vi "test-traj-generate-8-way.vi"() -> ()   [LabVIEW 2019]
uses:
  <vilib>/Rock Robotics/WPI/ThirdParty/JAS_Junk/TrajLib/WAYPOINTS.ctl
  <vilib>/Rock Robotics/WPI/ThirdParty/JAS_Junk/TrajLib/TRANSLATION2D.ctl
  <vilib>/Rock Robotics/WPI/ThirdParty/JAS_Junk/TrajLib/TRAJECTORY.ctl
  <vilib>/Rock Robotics/WPI/ThirdParty/JAS_Junk/TrajLib/TRAJ_STATE.ctl
  <vilib>/Rock Robotics/WPI/ThirdParty/JAS_Junk/TrajLib/POSE2D.ctl
  <vilib>/Rock Robotics/WPI/ThirdParty/JAS_Junk/TrajLib/ROTATION2D.ctl
  <vilib>/Rock Robotics/WPI/ThirdParty/JAS_Junk/TrajLib/X_Y_HEADING.ctl
  <vilib>/Rock Robotics/WPI/ThirdParty/JAS_Junk/TrajLib/SPLINE.ctl
  <vilib>/Analysis/Matrix/Datatypes/RealMatrix.ctl
  <vilib>/Rock Robotics/WPI/ThirdParty/JAS_Junk/TrajLib/POSEwCURVATURE.ctl
  <vilib>/Rock Robotics/WPI/ThirdParty/JAS_Junk/TrajLib/TRAJ_CONFIG.ctl
  <vilib>/Rock Robotics/WPI/ThirdParty/JAS_Junk/TrajLib/TRAJ_CONSTRAINT_DIIF_DRIVE_KINEMATICS.ctl
  <vilib>/Rock Robotics/WPI/ThirdParty/JAS_Junk/TrajLib/DIFF_DRIVE_KINEMATICS.ctl
  <vilib>/Rock Robotics/WPI/ThirdParty/JAS_Junk/TrajLib/TRAJ_CONSTRAINT_CENTRIPETAL_ACCEL.ctl
  <vilib>/Rock Robotics/WPI/ThirdParty/JAS_Junk/TrajLib/TRAJ_CONSTRAINT_SWERVE_DRIVE_KINEMATICS.ctl
  <vilib>/Rock Robotics/WPI/ThirdParty/JAS_Junk/TrajLib/SWERVE_DRIVE_KINEMATICS.ctl
  <vilib>/Rock Robotics/WPI/ThirdParty/JAS_Junk/TrajLib/TRAJ_CONSTRAINT_DIIF_DRIVE_VOLTAGE.ctl
  <vilib>/Rock Robotics/WPI/ThirdParty/JAS_Junk/TrajLib/SIMPLE_MOTOR_FF.ctl
  <vilib>/Rock Robotics/WPI/ThirdParty/JAS_Junk/TrajLib/TRAJ_CONSTRAINT_MECA_DRIVE_KINEMATICS.ctl
  <vilib>/Rock Robotics/WPI/ThirdParty/JAS_Junk/TrajLib/MECA_DRIVE_KINEMATICS.ctl
  <vilib>/Rock Robotics/WPI/ThirdParty/JAS_Junk/TrajLib/UTIL_WAYPOINT.ctl
  <vilib>/Rock Robotics/SystemInterfaces/NetworkCommunication/NetComm_UsageReport_report.vi
  <vilib>/Rock Robotics/WPI/ThirdParty/JAS_Junk/TrajLib/DiffDriveKinematicsConstraint_New.vi
  <vilib>/Rock Robotics/WPI/ThirdParty/JAS_Junk/TrajLib/CentripetalAccelConstraint_New.vi
  <vilib>/Rock Robotics/WPI/ThirdParty/JAS_Junk/TrajLib/Rotation_CreateAngle.vi
  <vilib>/Rock Robotics/WPI/ThirdParty/JAS_Junk/TrajLib/Translation_Create.vi
  <vilib>/Rock Robotics/WPI/ThirdParty/JAS_Junk/TrajLib/Util_LibraryGlobals.vi
  <vilib>/Rock Robotics/WPI/ThirdParty/JAS_Junk/TrajLib/Trajectory_Library.lvlib
  <vilib>/Analysis/Matrix/NI_Matrix.lvlib
panel:
  in  "Tab Control":T1(tab)
  in  "Interior WAYPOINTS":T2=[{"X"=1.5, "Y"=1.5}, {"X"=0.0, "Y"=0.0}, {"X"=-1.5, "Y"=-1.5}, {"X"=-3.0, "Y"=0.0}, {"X"=-1.5, "Y"=1.5}, {"X"=0.0, "Y"=0.0}, {"X"=1.5, "Y"=-1.5}]
  in  "Initial_Position":T4={"X"=3.0, "Y"=0.0, "Heading"=1.571}
  in  "Ending_Position":T4={"X"=3.0, "Y"=0.0, "Heading"=1.571}
  out "splines":T5[](array[typedef])
  out "ArrayPoseWithCurvature":T7[](array[typedef])
  out "PoseCSize":i32
  out "error out 2":errorcluster
  in  "MaxVelocity":dbl=2.0 format="%17.4f"
  in  "MaxAcceleration":dbl=1.3 format="%17.4f"
  in  "TrackWidth_Meters":dbl=0.66 format="%20.4f"
  in  "Max Cent Accel":dbl=1.0 format="%20.4f"
  out "outTRAJECTORY_CONFIG":T10={"MaxVelocity"=0.0, "Max Acceleration"=0.0, "StartVelocity"=0.0, "End Velocity"=0.0, "Reversed"=FALSE, "DiffDrKineConstntDefined"=FALSE, "CentAcellConstntDefined"=FALSE, "DiffDrVoltConstntDefined"=FALSE, "DIFF_DRIVE_KINE_CONSTRAINT"={"Max Speed (M/S)"=0.0, "DIFF_DRIVE_KINEMATICS"={"TrackWidth_Meters"=0.0}}, "CENTRIPETAL_ACCEL_CONSTRAINT"={"Max Cent Accel"=0.0}, "SwerveDrKineConstntDefined"=FALSE, "SWERVE_DRIVE_KINE_CONSTRAINT"={"Max Speed (M/S)"=0.0, "SwerveKinematics"={"NumModules"=0, "InverseKinematics"=[], "ForwardKinematics"=[], "Modules"=[], "PrevCoR"={"X"=0.0, "Y"=0.0}}}, "DIFF_DRIVE_VOLTAGE_CONSTRAINT"={"Max Voltage"=0.0, "DIFF_DRIVE_KINEMATICS"={"TrackWidth_Meters"=0.0}, "SIMPLE_MOTOR_FF"={"Ks"=0.0, "Kv"=0.0, "Ka"=0.0}}, "MECANUM_DRIVE_KINE_CONSTRAINT"={"Max Speed (M/S)"=0.0, "MECA_DRIVE_KINEMATICS"={"FrontLeft"={"X"=0.0, "Y"=0.0}, "FrontRight"={"X"=0.0, "Y"=0.0}, "RearLeft"={"X"=0.0, "Y"=0.0}, "RearRight"={"X"=0.0, "Y"=0.0}, "InverseKinematics"=[[0.0, 1.0, -1.0, 0.0], [0.0, 1.0, 1.0, 0.0], [0.0, 1.0, 1.0, 0.0], [0.0, 1.0, -1.0, 0.0]], "ForwardKinematics"=[[0.0, 1.0, -1.0, 0.0], [0.0, 1.0, 1.0, 0.0], [0.0, 1.0, 1.0, 0.0], [0.0, 1.0, -1.0, 0.0]], "PrevCoR"={"X"=0.0, "Y"=0.0}}}, "MecanumDrKineConstntDefined"=FALSE} {"MECANUM_DRIVE_KINE_CONSTRAINT"."MECA_DRIVE_KINEMATICS"."PrevCoR"."Y" format="%14.3f"; "MECANUM_DRIVE_KINE_CONSTRAINT"."MECA_DRIVE_KINEMATICS"."PrevCoR"."X" format="%14.3f"; "MECANUM_DRIVE_KINE_CONSTRAINT"."MECA_DRIVE_KINEMATICS"."RearRight"."Y" format="%14.3f"; "MECANUM_DRIVE_KINE_CONSTRAINT"."MECA_DRIVE_KINEMATICS"."RearRight"."X" format="%14.3f"; "MECANUM_DRIVE_KINE_CONSTRAINT"."MECA_DRIVE_KINEMATICS"."RearLeft"."Y" format="%14.3f"; "MECANUM_DRIVE_KINE_CONSTRAINT"."MECA_DRIVE_KINEMATICS"."RearLeft"."X" format="%14.3f"; "MECANUM_DRIVE_KINE_CONSTRAINT"."MECA_DRIVE_KINEMATICS"."FrontRight"."Y" format="%14.3f"; "MECANUM_DRIVE_KINE_CONSTRAINT"."MECA_DRIVE_KINEMATICS"."FrontRight"."X" format="%14.3f"; "MECANUM_DRIVE_KINE_CONSTRAINT"."MECA_DRIVE_KINEMATICS"."FrontLeft"."Y" format="%14.3f"; "MECANUM_DRIVE_KINE_CONSTRAINT"."MECA_DRIVE_KINEMATICS"."FrontLeft"."X" format="%14.3f"; "MECANUM_DRIVE_KINE_CONSTRAINT"."Max Speed (M/S)" format="%20.4f"; "DIFF_DRIVE_VOLTAGE_CONSTRAINT"."SIMPLE_MOTOR_FF"."Ka" format="%13.4f"; "DIFF_DRIVE_VOLTAGE_CONSTRAINT"."SIMPLE_MOTOR_FF"."Kv" format="%13.4f"; "DIFF_DRIVE_VOLTAGE_CONSTRAINT"."SIMPLE_MOTOR_FF"."Ks" format="%13.4f"; "DIFF_DRIVE_VOLTAGE_CONSTRAINT"."DIFF_DRIVE_KINEMATICS"."TrackWidth_Meters" format="%20.4f"; "DIFF_DRIVE_VOLTAGE_CONSTRAINT"."Max Voltage" format="%20.4f"; "SWERVE_DRIVE_KINE_CONSTRAINT"."SwerveKinematics"."PrevCoR"."Y" format="%14.3f"; "SWERVE_DRIVE_KINE_CONSTRAINT"."SwerveKinematics"."PrevCoR"."X" format="%14.3f"; "SWERVE_DRIVE_KINE_CONSTRAINT"."SwerveKinematics"."Modules"."Y" format="%14.3f"; "SWERVE_DRIVE_KINE_CONSTRAINT"."SwerveKinematics"."Modules"."X" format="%14.3f"; "SWERVE_DRIVE_KINE_CONSTRAINT"."Max Speed (M/S)" format="%20.4f"; "CENTRIPETAL_ACCEL_CONSTRAINT"."Max Cent Accel" format="%20.4f"; "DIFF_DRIVE_KINE_CONSTRAINT"."DIFF_DRIVE_KINEMATICS"."TrackWidth_Meters" format="%20.4f"; "DIFF_DRIVE_KINE_CONSTRAINT"."Max Speed (M/S)" format="%20.4f"; "End Velocity" format="%20.4f"; "StartVelocity" format="%20.4f"; "Max Acceleration" format="%20.4f"; "MaxVelocity" format="%20.4f"}
  out "TRAJECTORY":T20 {"TotalTImeSecs" format="%20.3f"}
  out "size(s)":i32
  out "error out":errorcluster
  out "read Traj":errorcluster
  out "readTRAJECTORY":T20 {"TotalTImeSecs" format="%20.3f"}
  out "size(s) 2":i32
  out "file write error":errorcluster
  out "appended path":path
  out "XY Graph":cluster{dbl[], dbl[]}(graph)
  out "Position":cluster{dbl[], dbl[]}(graph)
  out "Time":dbl
  in  "STEP":bool
  out "XY Graph 2":cluster{dbl[], dbl[]}(graph)
  out "TimeSeconds":dbl
  out "OutputTRAJ_STATE":T21={"TimeSeconds"=0.0, "Velocity"=0.0, "Acceleration"=0.0, "POSE"={"TRANSLATION"={"X"=0.0, "Y"=0.0}, "ROTATION"={"VALUE"=0.0, "COS"=1.0, "SIN"=0.0}}, "Curvature"=0.0}
  in  "CONT":bool
  out "Done":bool
  # "ARRAY OF OTHER\nCONSTRAINTS \nGOES HERE.."
  # "Single step\nthrough \ntrajectory"
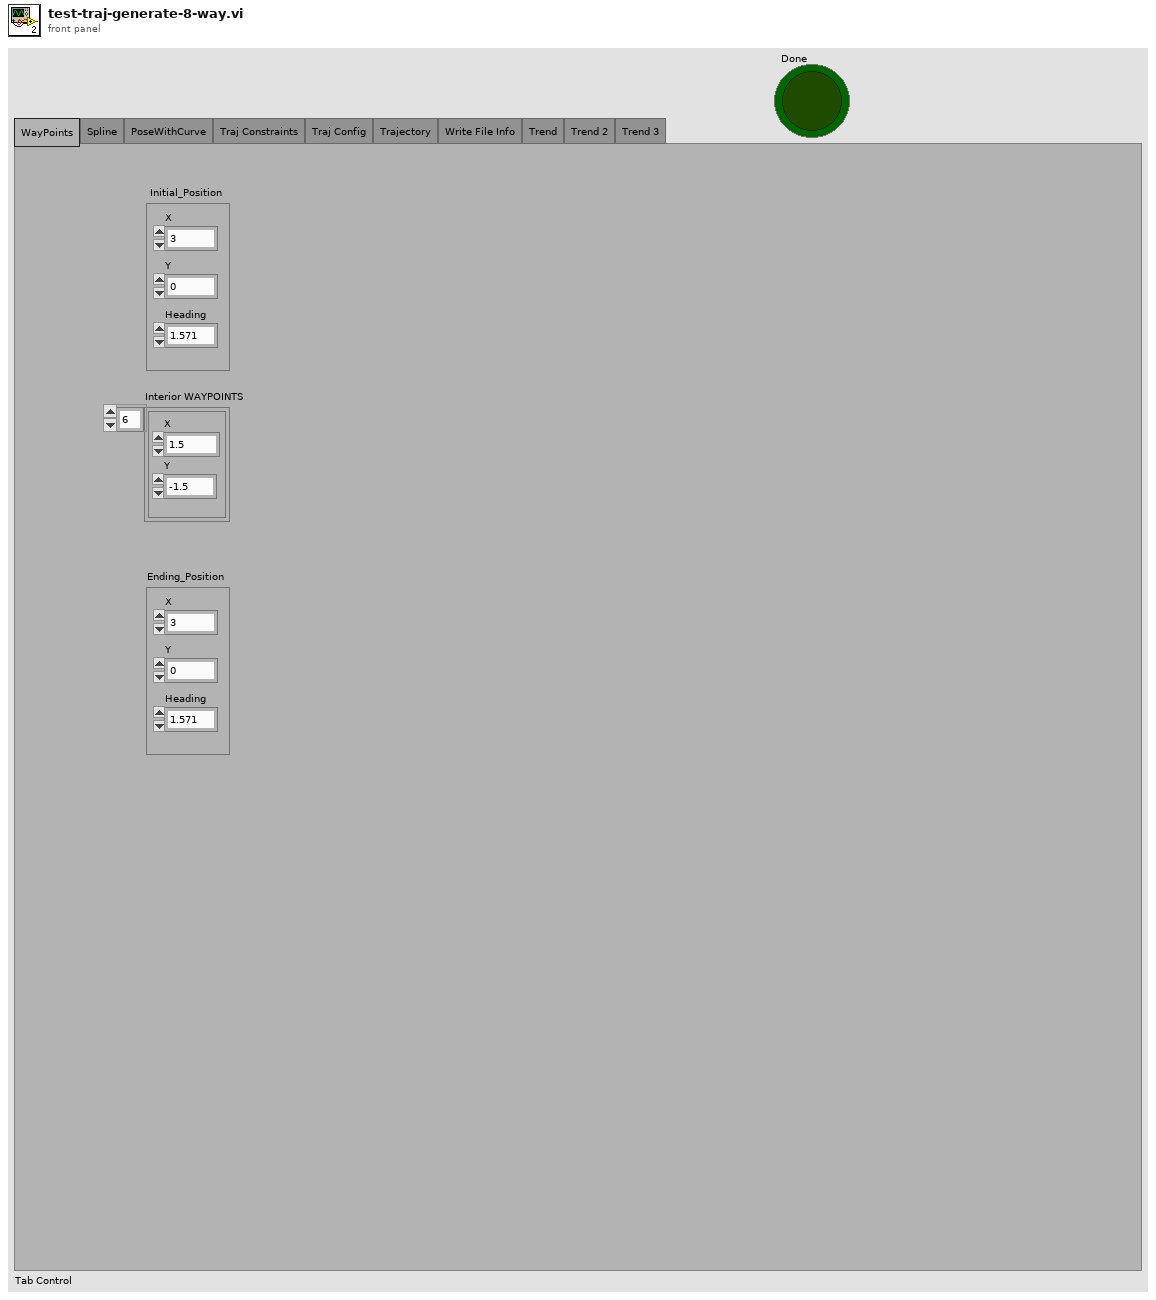
[diagram p1: front panel]
types:
  T1 = enum32{"WayPoints", "Spline", "PoseWithCurve", "Traj Constraints", "Traj Config", "Trajectory", "Write File Info", "Trend", "Trend 2", "Trend 3"}
  T2 = typedef "Trajectory_Library.lvlib/WAYPOINTS.ctl" = T3[]
  T3 = typedef "Trajectory_Library.lvlib/TRANSLATION2D.ctl" = cluster{"X":dbl, "Y":dbl}
  T4 = typedef "Trajectory_Library.lvlib/X_Y_HEADING.ctl" = cluster{"X":dbl, "Y":dbl, "Heading":dbl}
  T5 = typedef "Trajectory_Library.lvlib/SPLINE.ctl" = cluster{"Degree":i32, "Coefficients":T6}
  T6 = typedef "NI_Matrix.lvlib/RealMatrix.ctl" = dbl[][]
  T7 = typedef "Trajectory_Library.lvlib/POSEwCURVATURE.ctl" = cluster{"CURVATURE":dbl, "POSE":T8}
  T8 = typedef "Trajectory_Library.lvlib/POSE2D.ctl" = cluster{"TRANSLATION":T3, "ROTATION":T9}
  T9 = typedef "Trajectory_Library.lvlib/ROTATION2D.ctl" = cluster{"VALUE":dbl, "COS":dbl, "SIN":dbl}
  T10 = typedef "Trajectory_Library.lvlib/TRAJ_CONFIG.ctl" = cluster{"MaxVelocity":dbl, "Max Acceleration":dbl, "StartVelocity":dbl, "End Velocity":dbl, "Reversed":bool, "DiffDrKineConstntDefined":bool, "CentAcellConstntDefined":bool, "DiffDrVoltConstntDefined":bool, "DIFF_DRIVE_KINE_CONSTRAINT":T11, "CENTRIPETAL_ACCEL_CONSTRAINT":T13, "SwerveDrKineConstntDefined":bool, "SWERVE_DRIVE_KINE_CONSTRAINT":T14, "DIFF_DRIVE_VOLTAGE_CONSTRAINT":T16, "MECANUM_DRIVE_KINE_CONSTRAINT":T18, "MecanumDrKineConstntDefined":bool}
  T11 = typedef "Trajectory_Library.lvlib/TRAJ_CONSTRAINT_DIIF_DRIVE_KINEMATICS.ctl" = cluster{"Max Speed (M/S)":dbl, "DIFF_DRIVE_KINEMATICS":T12}
  T12 = typedef "Trajectory_Library.lvlib/DIFF_DRIVE_KINEMATICS.ctl" = cluster{"TrackWidth_Meters":dbl}
  T13 = typedef "Trajectory_Library.lvlib/TRAJ_CONSTRAINT_CENTRIPETAL_ACCEL.ctl" = cluster{"Max Cent Accel":dbl}
  T14 = typedef "Trajectory_Library.lvlib/TRAJ_CONSTRAINT_SWERVE_DRIVE_KINEMATICS.ctl" = cluster{"Max Speed (M/S)":dbl, "SwerveKinematics":T15}
  T15 = typedef "Trajectory_Library.lvlib/SWERVE_DRIVE_KINEMATICS.ctl" = cluster{"NumModules":i32, "InverseKinematics":T6, "ForwardKinematics":T6, "Modules":T3[], "PrevCoR":T3}
  T16 = typedef "Trajectory_Library.lvlib/TRAJ_CONSTRAINT_DIIF_DRIVE_VOLTAGE.ctl" = cluster{"Max Voltage":dbl, "DIFF_DRIVE_KINEMATICS":T12, "SIMPLE_MOTOR_FF":T17}
  T17 = typedef "Trajectory_Library.lvlib/SIMPLE_MOTOR_FF.ctl" = cluster{"Ks":dbl, "Kv":dbl, "Ka":dbl}
  T18 = typedef "Trajectory_Library.lvlib/TRAJ_CONSTRAINT_MECA_DRIVE_KINEMATICS.ctl" = cluster{"Max Speed (M/S)":dbl, "MECA_DRIVE_KINEMATICS":T19}
  T19 = typedef "Trajectory_Library.lvlib/MECA_DRIVE_KINEMATICS.ctl" = cluster{"FrontLeft":T3, "FrontRight":T3, "RearLeft":T3, "RearRight":T3, "InverseKinematics":T6, "ForwardKinematics":T6, "PrevCoR":T3}
  T20 = typedef "Trajectory_Library.lvlib/TRAJECTORY.ctl" = cluster{"TotalTImeSecs":dbl, "States":T21[]}
  T21 = typedef "Trajectory_Library.lvlib/TRAJ_STATE.ctl" = cluster{"TimeSeconds":dbl, "Velocity":dbl, "Acceleration":dbl, "POSE":T8, "Curvature":dbl}
  T22 = typedef "Trajectory_Library.lvlib/UTIL_WAYPOINT.ctl" = cluster{"X":dbl, "Y":dbl, "ANGLE":dbl}
  T23 = typedef "Trajectory_Library.lvlib/SPLINE_CTRL_VECTOR.ctl" = cluster{"Xs":dbl[], "Ys":dbl[]}
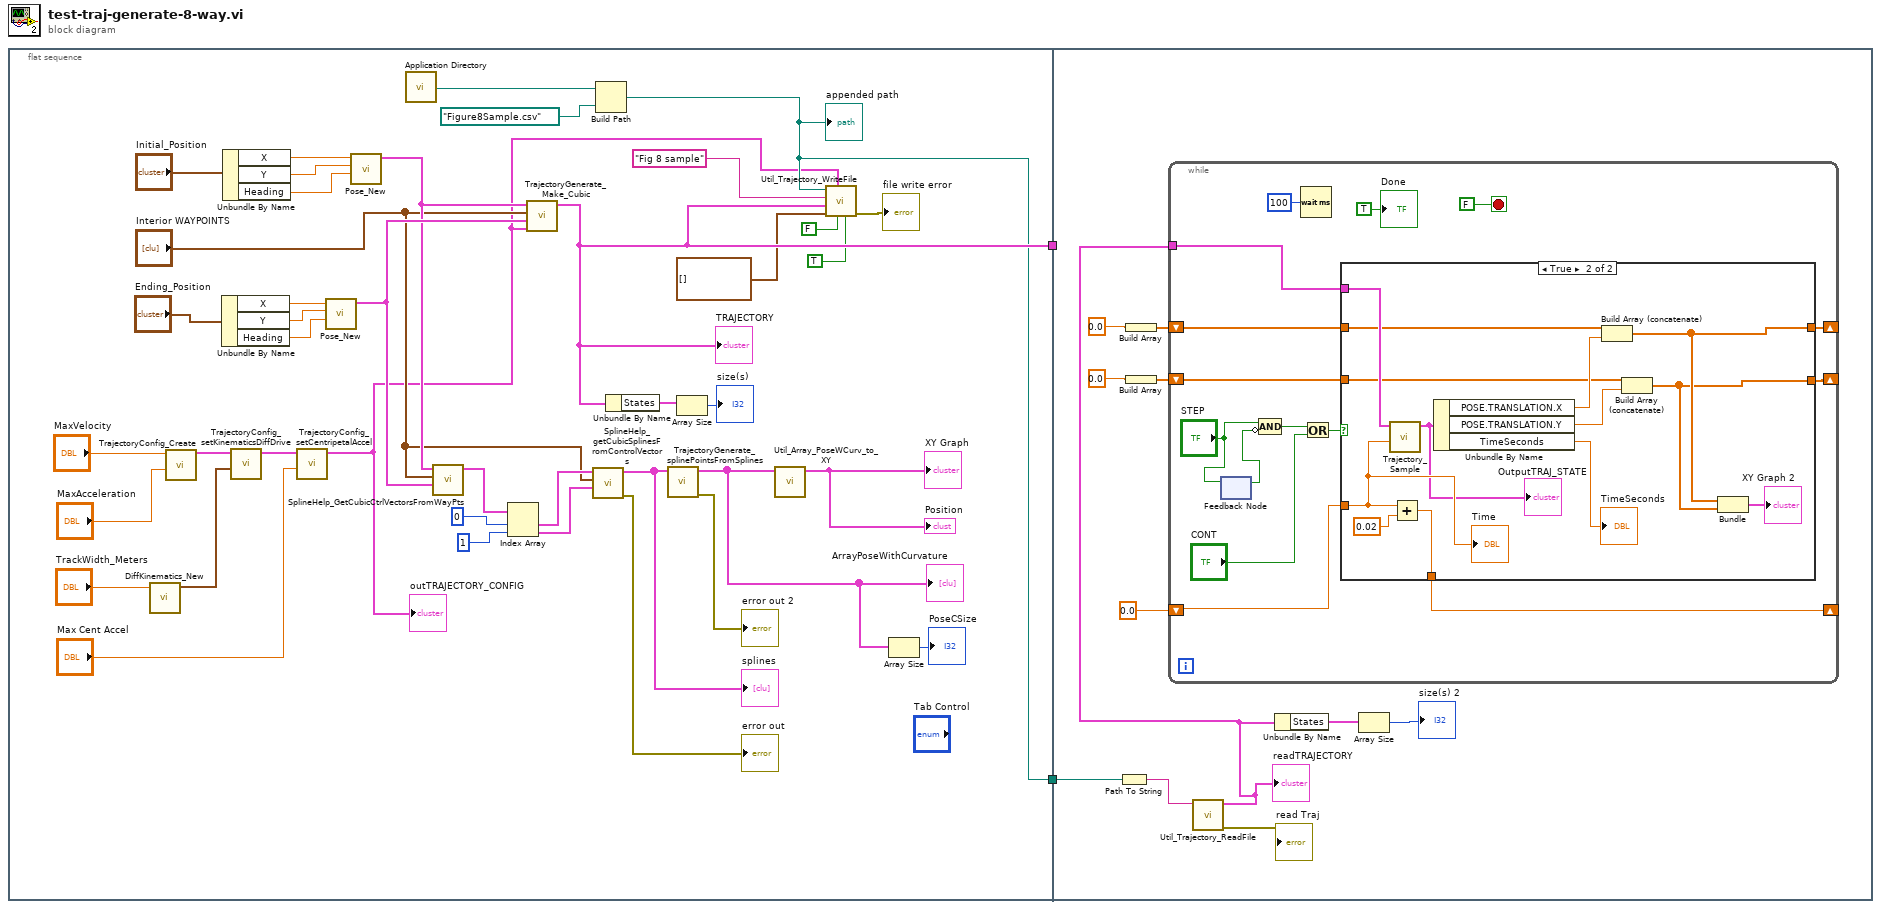
[diagram p0: block diagram]
diagram:
  n1 = flat-sequence {
    tunnel: [w21] -> w2
    tunnel: [w9] -> w1
    tunnel: w2 -> [_]
    tunnel: w1 -> [w47]
    frame #0 {
      n2 = call <vilib>:"DiffKinematics_New.vi"("TrackWidth_Meters"="TrackWidth_Meters") -> ("DIFF_DRIVE_KINEMATICS"=w14:T12)  [unwired: 10 in]
      n3 = call <vilib>:"TrajectoryConfig_Create.vi"("MaxAcceleration"="MaxAcceleration", "MaxVelocity"="MaxVelocity") -> ("TRAJECTORY_CONFIG"=w16:T10)  [unwired: 9 in]
      n4 = Unbundle By Name("Ending_Position") -> ("X"=w39:dbl, "Y"=w38:dbl, "Heading"=w37:dbl)
      n5 = Unbundle By Name("Initial_Position") -> ("X"=w42:dbl, "Y"=w41:dbl, "Heading"=w40:dbl)
      n6 = call <vilib>:"TrajectoryConfig_setKinematicsDiffDrive.vi"("DIFF_DRIVE_KINEMATICS"=w14, "inTRAJECTORY_CONFIG"=w16) -> ("outTRAJECTORY_CONFIG"=w13:T10)  [unwired: 9 in]
      n7 = call <vilib>:"TrajectoryConfig_setCentripetalAccel.vi"("Max Cent Accel"="Max Cent Accel", "inTRAJECTORY_CONFIG"=w13) -> ("outTRAJECTORY_CONFIG"=w7:T10)  [unwired: 9 in]
      "outTRAJECTORY_CONFIG" <- w7
      n8 = call <vilib>:"Pose_New.vi"("Heading"=w37, "Y"=w38, "X"=w39) -> ("out POSe"=w35:T8)  [unwired: 8 in]
      n9 = call <vilib>:"Pose_New.vi"("Heading"=w40, "Y"=w41, "X"=w42) -> ("out POSe"=w34:T8)  [unwired: 8 in]
      n10 = call <vilib>:"Application Directory.vi"() -> ("Application Directory"=w10:path)
      n11 = call <vilib>:"SplineHelp_GetCubicCtrlVectorsFromWayPts.vi"("Enging POSE"=w35, "Interior WAYPOINTS"="Interior WAYPOINTS", "Starting POSE"=w34) -> ("SplineControlVectors"=w24:T23[])  [unwired: 8 in]
      n12 = Index Array(array=w24, index #1=0 ("index"), index #2=1 ("index")) -> (element #1=w23:T23, element #2=w22:T23)
      n13 = call <vilib>:"TrajectoryGenerate_Make_Cubic.vi"("traj_config"=w7, "Enging POSE"=w35, "Interior WAYPOINTS"="Interior WAYPOINTS", "Starting POSE"=w34) -> ("TRAJECTORY"=w21:T20)  [unwired: 6 in, 1 out]
      "TRAJECTORY" <- w21
      n14 = call <vilib>:"SplineHelp_getCubicSplinesFromControlVectors.vi"("endCtrlVector"=w22, "InternalWaypoints"="Interior WAYPOINTS", "startCtrlVector"=w23) -> ("error out"=→"error out":errorcluster, "splines"=w32:T5[])  [unwired: 3 in, 4 out]
      "splines" <- w32
      n15 = Build Path(base path=w10, name or relative path=path "Figure8Sample.csv" ("Trajectory File Name")) -> (appended path=w9:path)
      "appended path" <- w9
      n16 = Unbundle By Name(w21) -> ("States"=w30:T21[])
      n17 = call <vilib>:"TrajectoryGenerate_splinePointsFromSplines.vi"("inputSPLINE"=w32) -> ("error out"=→"error out 2":errorcluster, "ArrayPoseWithCurvature"=w5:T7[])  [unwired: 9 in]
      "ArrayPoseWithCurvature" <- w5
      n18 = Array Size(array=w30) -> (size(s)=→"size(s)":i32)
      n19 = call <vilib>:"Util_Array_PoseWCurv_to_XY.vi"("inArrayPoseWCurve"=w5) -> ("outArrayXY"=→"XY Graph" →"Position":cluster{dbl[], dbl[]})  [unwired: 10 in]
      n20 = call <vilib>:"Util_Trajectory_WriteFile.vi"("Trajectory is Cubic"=TRUE, "Trajectory Is Relative"=FALSE, "TRAJECTORY_CONFIG"=w7, "UtilityWayPoints"=T22[] [], "TRAJECTORY"=w21, "Comment"="Fig 8 sample", "Trajectory File Name"=w9) -> ("error out"=→"file write error":errorcluster)  [unwired: 4 in]
      n21 = Array Size(array=w5) -> (size(s)=→"PoseCSize":i32)
    }
    frame #1 {
      n22 = Path To String(path=w47) -> (string=w48:string)
      n23 = Build Array(0.0) -> (w51:dbl[])
      n24 = Build Array(0.0) -> (w50:dbl[])
      n25 = call <vilib>:"Util_Trajectory_ReadFile.vi"("FileName"=w48) -> ("error out"=→"read Traj":errorcluster, "outTRAJECTORY"=w44:T20)  [unwired: 9 in]
      "readTRAJECTORY" <- w44
      n26 = while {
        shift-right: [w65] -> _
        shift-left: 0.0 -> [w66]
        tunnel: w44 -> [w62]
        shift-right: [w61] -> _
        shift-left: w51 -> [w64]
        shift-right: [w60] -> _
        shift-left: w50 -> [w63]
        stop <- FALSE stop-if-true
        n27 = feedback-in #1("STEP") -> ()
        n28 = feedback #1() -> (w58:bool)  [unwired: 1 in]
        n29 = Compound Arithmetic op=AND("STEP", invert w58) -> (w56:bool)
        n30 = Wait (ms)(milliseconds to wait=u32 100) -> ()  [unwired: 1 out]
        n31 = Or(x=w56, y="CONT") -> (x .or. y?=w57:bool)
        n32 = case shown="True" w57 {
          tunnel: w66 -> [w72 w83]
          tunnel: [w72 w85] -> w65
          tunnel: w64 -> [w71 w79]
          tunnel: w63 -> [w70 w77]
          tunnel: w62 -> [_ w82]
          tunnel: [w71 w74] -> w61
          tunnel: [w70 w73] -> w60
          frame False {
          }
          frame True {
            n33 = call <vilib>:"Trajectory_Sample.vi"("Time"=w83, "InputTRAJECTORY"=w82) -> ("OutputTRAJ_STATE"=w81:T21)  [unwired: 9 in]
            "OutputTRAJ_STATE" <- w81
            n34 = Add(x=w83, y=0.02) -> (x+y=w85:dbl)
            n35 = Unbundle By Name(w81) -> ("POSE.TRANSLATION.X"=w78:dbl, "POSE.TRANSLATION.Y"=w76:dbl, "TimeSeconds"=→"TimeSeconds":dbl)
            n36 = Build Array (concatenate)(w79, w78) -> (w74:dbl[])
            n37 = Build Array (concatenate)(w77, w76) -> (w73:dbl[])
            n38 = Bundle(w74, w73) -> (→"XY Graph 2":cluster{dbl[], dbl[]})  [unwired: 1 in]
            "Time" <- w83
          }
        }
        "Done" <- TRUE ("Done")
      }
      n39 = Unbundle By Name(w44) -> ("States"=w46:T21[])
      n40 = Array Size(array=w46) -> (size(s)=→"size(s) 2":i32)
    }
  }
